vi "testing_fpga.vi"() -> ()   [LabVIEW 2015]
uses:
  <vilib>/FPGAPlugInAG/myRIO-1900/niLvFpga_Open_myRIO-1900.vi
  <vilib>/rvi/interface/common/dynamic/niFpgaDynamicAddResources.vi
  <vilib>/Utility/error.llb/Error Cluster From Error Code.vi
  <vilib>/rvi/errors/niLvFpgaAdjustHostInterfaceError.vi
  <vilib>/FPGAPlugInAG/Dynamic/niLvFpga_Close_Dynamic.vi
  <vilib>/rvi/interface/nirviOpenFPGA/nirviOpenFPGA.xnode
  FPGA Bitfiles/Milestone4_FPGATarget_FPGAReadRightSen_eF1uKYxttK0.lvbitx
  physical_robot/FPGA Read Right Sensor.vi
  FPGA Bitfiles/Milestone4_FPGATarget_FPGAReadBackSens_nBWPgGusvV4.lvbitx
  physical_robot/FPGA Read Back Sensor.vi
  <vilib>/rvi/interface/nirviReadWriteControl/nirviReadWriteControl.xnode
  <vilib>/rvi/interface/nirviCloseFPGA/nirviCloseFPGA.xnode
  NiFpgaLv.dll
  <vilib>/rvi/interface/Simulation/niFpgaSimulationCallBeginRW.vi
panel:
  out "Time of Flight 2":u32
  out "Time of Flight":u32
  in  "stop":bool
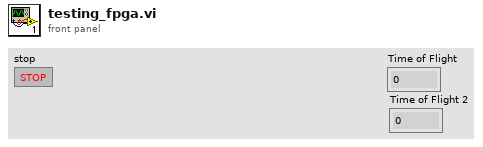
[diagram p1: front panel]
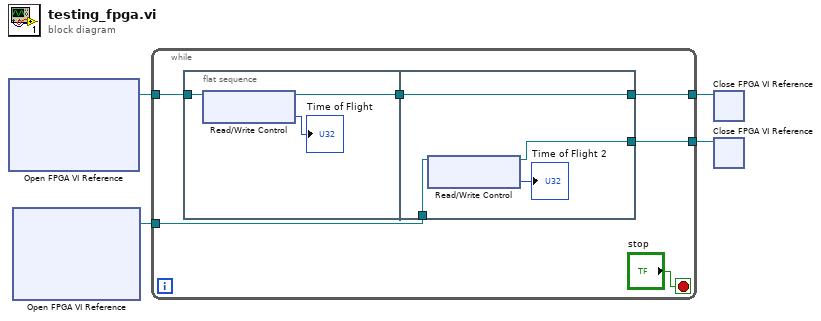
[diagram p0: block diagram]
diagram:
  n1 = xnode "Open FPGA VI Reference"() -> ("FPGA VI Reference Out"=w4:refnum<k20>)  [unwired: 2 in, 1 out]
  n2 = xnode "Open FPGA VI Reference"() -> ("FPGA VI Reference Out"=w2:refnum<k20>)  [unwired: 2 in, 1 out]
  n3 = while {
    tunnel: w4 -> [w10]
    tunnel: [w8] -> w3
    tunnel: w2 -> [w6]
    tunnel: [w5] -> w1
    stop <- "stop" stop-if-true
    n4 = flat-sequence {
      tunnel: w10 -> [w13]
      tunnel: [w11] -> w7
      tunnel: [w17] -> w8
      tunnel: w7 -> [w17]
      tunnel: w6 -> [w15]
      tunnel: [w14] -> w5
      frame #0 {
        n5 = xnode "Read/Write Control"("FPGA VI Reference In"=w13) -> ("FPGA VI Reference Out"=w11:refnum<k20>, "Time of Flight"=→"Time of Flight":u32)  [unwired: 1 in, 1 out]
      }
      frame #1 {
        n6 = xnode "Read/Write Control"("FPGA VI Reference In"=w15) -> ("FPGA VI Reference Out"=w14:refnum<k20>, "Time of Flight"=→"Time of Flight 2":u32)  [unwired: 1 in, 1 out]
      }
    }
  }
  n7 = xnode "Close FPGA VI Reference"("FPGA VI Reference In"=w3) -> ()  [unwired: 1 in, 1 out]
  n8 = xnode "Close FPGA VI Reference"("FPGA VI Reference In"=w1) -> ()  [unwired: 1 in, 1 out]
